vi "2 DirectionChangeGoodness.vi"(1 "Test Heading":dbl=57.0) -> (0 "Goodness":dbl=0.027051846866350416)   [LabVIEW 2011]
doc: "The DirectionChangeGoodness VI outputs a value between 1 and 0 that represents the goodness of the hypothetical heading from the perspective of turning as little as possible."
uses:
  2 Typedefs/heading.ctl
  2 Globals/2 Global.vi
  2 Globals/2 TuningConstants.vi
panel:
  out "Wind Adjustment":dbl=0.2
  in  "Tuning Quotient":i32=60
  out "Current Heading":T1 format="%05.1f"
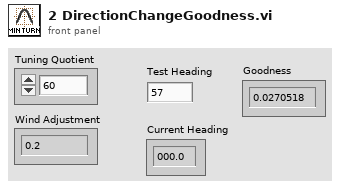
[diagram p1: front panel]
types:
  T1 = typedef "heading.ctl" = dbl
  T2 = typedef "apparent wind.ctl" = cluster{"Toward Fore":dbl, "Toward Starboard":dbl}
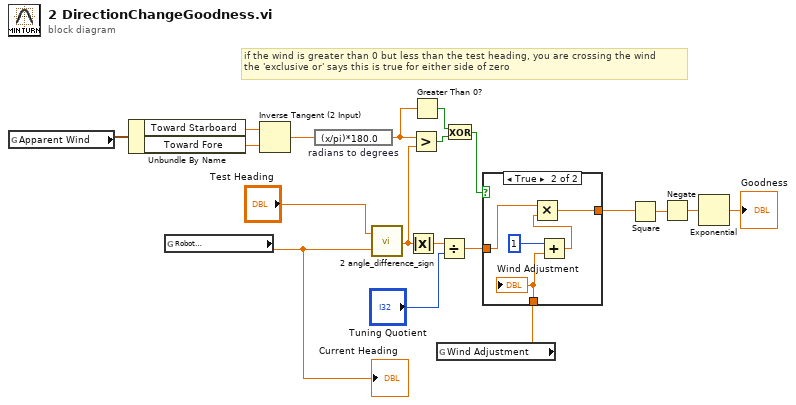
[diagram p0: block diagram]
diagram:
  # "if the wind is greater than 0 but less than the test heading, you are crossing the wind\nthe 'exclusive or' says this is true for either side of zero"
  n1 = global read "2 Global.vi" "Apparent Wind"() -> (w11:T2)
  n2 = Unbundle By Name(w11) -> ("Toward Starboard"=w8:dbl, "Toward Fore"=w7:dbl)
  n3 = global read "2 Global.vi" "Robot\nHeading"() -> (w15:T1)
  "Current Heading" <- w15
  n4 = Inverse Tangent (2 Input)(1:w7, 2:w8) -> (0:w2:dbl)
  n5 = expression code="(x/pi)*180.0" "radians to degrees"(w2) -> (w5:dbl)
  n6 = call "2 angle_difference_sign.vi"("Angle 2"=w15, "Angle 1"="Test Heading") -> ("Difference"=w6:dbl)
  n7 = Absolute Value(x=w6) -> (abs(x)=w10:dbl)
  n8 = Greater?(x=w5, y=w6) -> (0:w4:bool)
  n9 = Greater Than 0?(x=w5) -> (x > 0?=w3:bool)
  n10 = global read "2 TuningConstants.vi" "Wind Adjustment"() -> (w1:dbl)
  n11 = Divide(x=w10, y="Tuning Quotient") -> (x/y=w13:dbl)
  n12 = Exclusive Or(1:w4, 2:w3) -> (0:w9:bool)
  n13 = case shown="True" w9 {
    tunnel: [w20 w24] -> w12
    tunnel: w13 -> [w20 w25]
    tunnel: w1 -> [_ w21]
    frame False {
    }
    frame True {
      n14 = Add(x=1, y=w21) -> (x+y=w22:dbl)
      n15 = Multiply(x=w25, y=w22) -> (x*y=w24:dbl)
      "Wind Adjustment" <- w21
    }
  }
  n16 = Square(x=w12) -> (x^2=w17:dbl)
  n17 = Negate(x=w17) -> (-x=w18:dbl)
  n18 = Exponential(1:w18) -> (0:→"Goodness":dbl)
